vi "_emi_Start Loop Single.vi"(2 "Start even on error(T)":bool=TRUE, 5 "Loop ID in":u16, 7 "Allow start(T)":bool=TRUE, 9 "error in (no error)":errorcluster) -> (6 "Loop ID out":u16, 10 "error out":errorcluster, 13 "Start loop":bool)   [LabVIEW 2010]
doc: "Check wheter a loop should start. based on loop enable(Loop control),\n\nExecutes as normal on error"
uses:
  _emi_Loop control int action.ctl
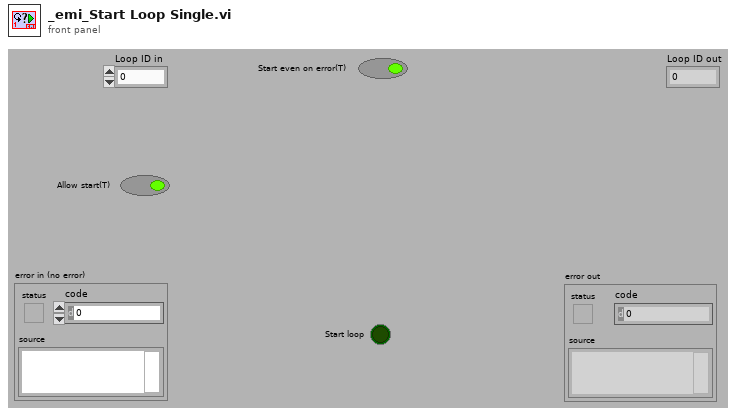
[diagram p1: front panel]
types:
  T1 = typedef "_emi_Loop control int action.ctl" = enum16{"Init index", "Get index", "Set index", "Get Size"}
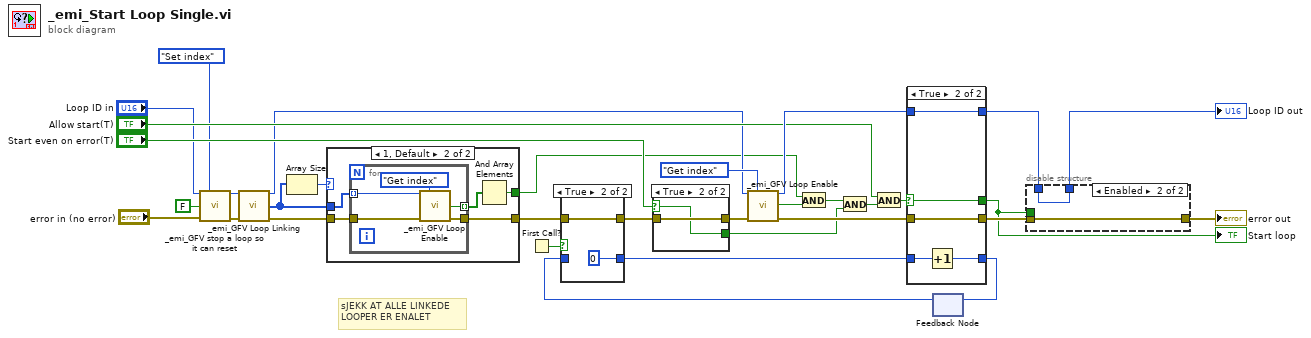
[diagram p0: block diagram]
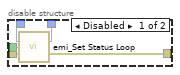
[diagram p2: hidden frame]
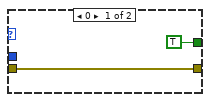
[diagram p3: hidden frame]
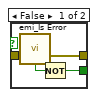
[diagram p4: hidden frame]
diagram:
  # "sJEKK AT ALLE LINKEDE\nLOOPER ER ENALET"
  n1 = call "_emi_GFV stop a loop so it can reset.vi"("Loop Index/Numb"="Loop ID in", "Action(Get Index)"=_emi_Loop_control_int_action."Set index", "Value In"=FALSE, "error in (no error)"="error in (no error)") -> ("Index out"=w8:u16, "error out"=w9:errorcluster)  [unwired: 8 in, 2 out]
  n2 = call "_emi_GFV Loop Linking.vi"("Loop Index/Numb"=w8, "error in (no error)"=w9) -> ("Index out"=w7:u16, "Linked indexes out"=w4:u16[], "error out"=w5:errorcluster)  [unwired: 10 in, 1 out]
  n3 = Array Size(array=w4) -> (size(s)=w6:i32)
  n4 = case shown="1, Default" w6 {
    tunnel: w5 -> [w34 w40]
    tunnel: w4 -> [_ w36]
    tunnel: [w34 w39] -> w3
    tunnel: [TRUE w37] -> w1
    frame 0 {
    }
    frame 1, Default {
      n5 = for {
        tunnel: w40 -> [w45]
        tunnel: [w44] -> w39
        tunnel: [w42] -> w38 mode=indexing
        tunnel: w36 -> [w41] mode=indexing
        n6 = call "_emi_GFV Loop Enable.vi"("Loop Index/Numb"=w41, "Action(Get Index)"=_emi_Loop_control_int_action."Get index", "error in (no error)"=w45) -> ("Loop Enable Out"=w42:bool, "error out"=w44:errorcluster)  [unwired: 9 in, 2 out]
      }
      n7 = And Array Elements(Boolean array=w38) -> (logical AND=w37:bool)
    }
  }
  n8 = First Call?() -> (First Call?: T/F=w33:bool)
  n9 = feedback #1() -> (w30:i32)  [unwired: 1 in]
  n10 = case shown="True" w33 {
    tunnel: [w47 w49] -> w29
    tunnel: w3 -> [w47 w49]
    tunnel: [w46 0] -> w31
    tunnel: w30 -> [w46 _]
    frame False {
    }
    frame True {
    }
  }
  n11 = case shown="True" "Start even on error(T)" {
    selector: "Start even on error(T)" -> [_ w54]
    tunnel: w29 -> [w53 w55]
    tunnel: [w52 w55] -> w27
    tunnel: [w51 w54] -> w22
    frame False {
      n12 = call "emi_Is Error.vi"("error in (no error)"=w53) -> ("error out"=w52:errorcluster, "Is Error"=w50:bool)  [unwired: 13 in]
      n13 = Not(x=w50) -> (.not. x?=w51:bool)
    }
    frame True {
    }
  }
  n14 = call "_emi_GFV Loop Enable.vi"("Loop Index/Numb"=w7, "Action(Get Index)"=_emi_Loop_control_int_action."Get index", "error in (no error)"=w27) -> ("Index out"=w24:u16, "Loop Enable Out"=w23:bool, "error out"=w26:errorcluster)  [unwired: 9 in, 1 out]
  n15 = And(x=w1, y=w23) -> (x .and. y?=w2:bool)
  n16 = And(x=w2, y=w22) -> (x .and. y?=w21:bool)
  n17 = And(x="Allow start(T)", y=w21) -> (x .and. y?=w15:bool)
  n18 = case shown="True" w15 {
    selector: w15 -> [w57 w62]
    tunnel: [w59 w64] -> w17
    tunnel: w24 -> [w59 w64]
    tunnel: [w58 w63] -> w20
    tunnel: w26 -> [w58 w63]
    tunnel: [w57 w62] -> w16
    tunnel: [w56 w60] -> w32
    tunnel: w31 -> [w56 w61]
    frame False {
    }
    frame True {
      n19 = Increment(x=w61) -> (x+1=w60:i32)
    }
  }
  "Start loop" <- w16
  n20 = feedback-in #1(w32) -> ()
  n21 = disable-structure shown="Enabled" {
    disable-tunnel: w20 -> [w69 w71]
    disable-tunnel: [w68 w71] -> w19
    disable-tunnel: [w67 w70] -> w18
    disable-tunnel: w17 -> [w66 w70]
    disable-tunnel: w16 -> [w65 _]
    frame Disabled {
      n22 = call "emi_Set Status Loop.vi"("Loop ID in"=w66, "Running?"=w65, "error in (no error)"=w69) -> ("Loop ID out"=w67:u16, "error out"=w68:errorcluster)  [unwired: 11 in]
    }
    frame Enabled {
    }
  }
  "error out" <- w19
  "Loop ID out" <- w18
